vi "Zadanie 1.vi"() -> ()   [LabVIEW 2020]
panel:
  out "Min":dbl
  out "Max":dbl
  out "RMS":dbl
  in  "Offset harmonicznej 2":dbl(knob) scale=0.0..10.0
  in  "Faza harmonicznej 2":dbl(knob) scale=0.0..10.0
  in  "Amplituda harmonicznej 2":dbl(knob) scale=0.0..10.0
  in  "Offset harmonicznej 1":dbl(knob) scale=0.0..10.0
  in  "Faza harmonicznej 1":dbl(knob) scale=0.0..10.0
  in  "Amplituda harmonicznej 1":dbl(knob) scale=0.0..10.0
  in  "2 harmoniczna":dbl
  in  "1 harmoniczna":dbl
  in  "Stop":bool
  in  "Czêstotliwoœæ":dbl(knob) scale=0.0..10.0
  in  "Offset":dbl(knob) scale=0.0..10.0
  in  "Faza":dbl(knob) scale=0.0..10.0
  in  "Amplituda":dbl(knob) scale=0.0..10.0
  out "Waveform Graph":dynamicdata(graph)
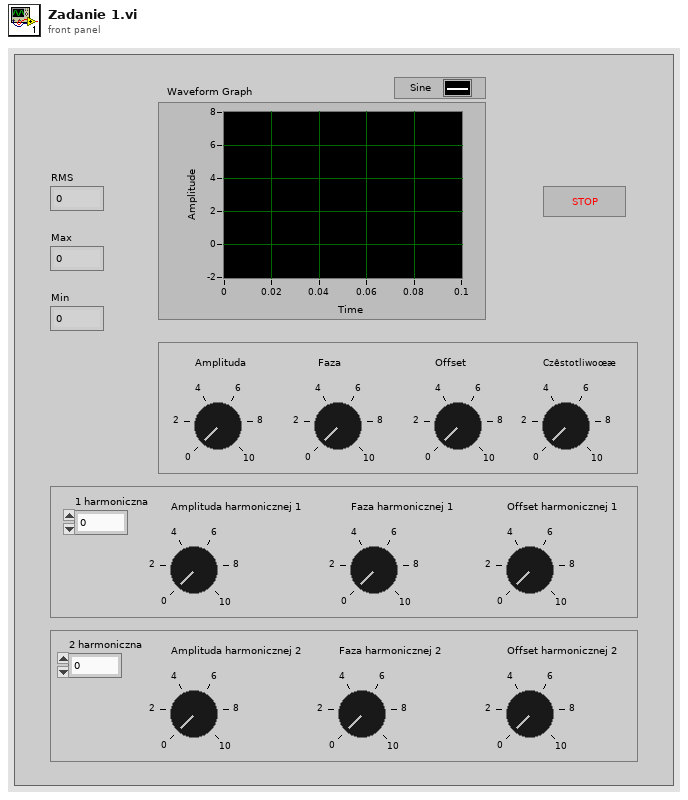
[diagram p1: front panel]
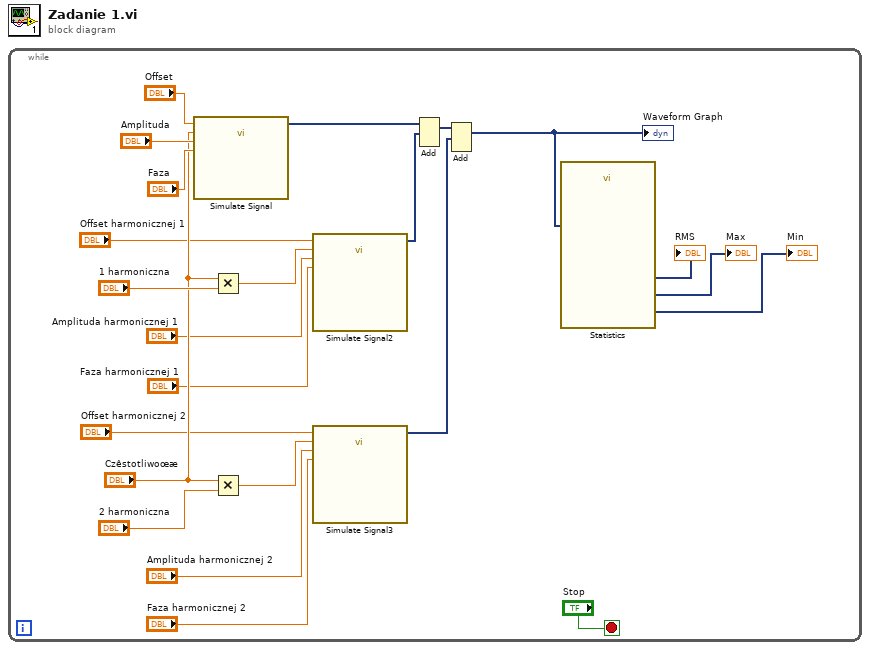
[diagram p0: block diagram]
diagram:
  n1 = while {
    stop <- "Stop" stop-if-true
    n2 = call "Simulate Signal"("Offset"="Offset", "Frequency"="Czêstotliwoœæ", "Amplitude"="Amplituda", "Phase"="Faza") -> ("Sine"=w14:dynamicdata)  [unwired: 10 in, 1 out]
    n3 = Multiply(x="Czêstotliwoœæ", y="1 harmoniczna") -> (x*y=w19:dbl)
    n4 = Multiply(x="Czêstotliwoœæ", y="2 harmoniczna") -> (x*y=w18:dbl)
    n5 = call "Simulate Signal2"("Offset"="Offset harmonicznej 1", "Frequency"=w19, "Amplitude"="Amplituda harmonicznej 1", "Phase"="Faza harmonicznej 1") -> ("Sine"=w13:dynamicdata)  [unwired: 10 in, 1 out]
    n6 = call "Simulate Signal3"("Offset"="Offset harmonicznej 2", "Frequency"=w18, "Amplitude"="Amplituda harmonicznej 2", "Phase"="Faza harmonicznej 2") -> ("Sine"=w11:dynamicdata)  [unwired: 10 in, 1 out]
    n7 = Add(1:w13, 2:w14) -> (0:w12:dynamicdata)  [unwired: 1 in, 1 out]
    n8 = Add(1:w11, 2:w12) -> (0:w4:dynamicdata)  [unwired: 1 in, 1 out]
    "Waveform Graph" <- w4
    n9 = call "Statistics"("Signals"=w4) -> ("RMS"=→"RMS":dynamicdata, "Minimum"=→"Min":dynamicdata, "Maximum"=→"Max":dynamicdata)  [unwired: 23 in, 1 out]
  }
